vi "save_dc_res.vi"(0 "current state":dbl, 1 "cell number":string, 2 "dc resistance":string, 3 "file path":path) -> ()   [LabVIEW 2016]
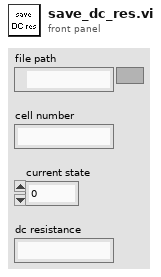
[diagram p1: front panel]
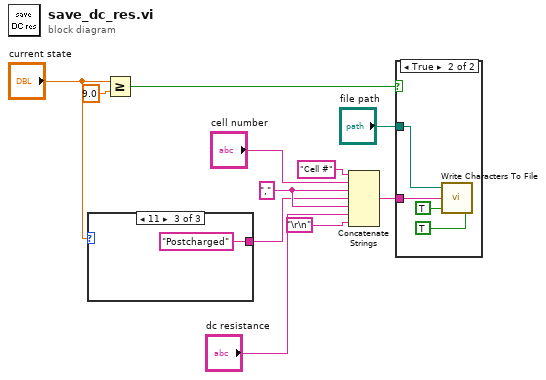
[diagram p0: block diagram]
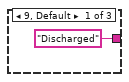
[diagram p2: hidden frame]
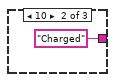
[diagram p3: hidden frame]
diagram:
  w10 = "," ("string")
  n1 = case shown="11" "current state" {
    tunnel: ["Discharged" "Charged" "Postcharged"] -> w1
    frame 9, Default {
    }
    frame 10 {
    }
    frame 11 {
    }
  }
  n2 = Greater Or Equal?(x="current state", y=9.0) -> (x >= y?=w7:bool)
  n3 = Concatenate Strings("Cell #" ("string"), "cell number", w10, w1, w10, "dc resistance", "\r\n") -> (w4:string)
  n4 = case shown="True" w7 {
    tunnel: w4 -> [_ w16]
    tunnel: "file path" -> [_ w15]
    frame False {
    }
    frame True {
      n5 = call <vilib>:"Write Characters To File.vi"("convert eol? (no:F)"=TRUE, "append to file? (new file:F)"=TRUE, "character string"=w16, "file path (dialog if empty)"=w15) -> ()  [unwired: 1 in, 1 out]
    }
  }
